vi "PH_Beckhoff_Application.declare digital PILS external OutputTags.vi"() -> (0 "Digital Outputs":T2, 1 "Description":string)   [LabVIEW 2014, in "PH_Beckhoff_Application.lvlib"]
uses:
  PH_Beckhoff_Application.lvlib
  PH_Beckhoff/PH_Beckhoff.Digital Outputs.ctl
  PH_Beckhoff/PH_Beckhoff.lvlib
panel:
  in  "Digital Output Value":T1
  out "Right Size?":bool
  # "Let this VI run to check the size!"
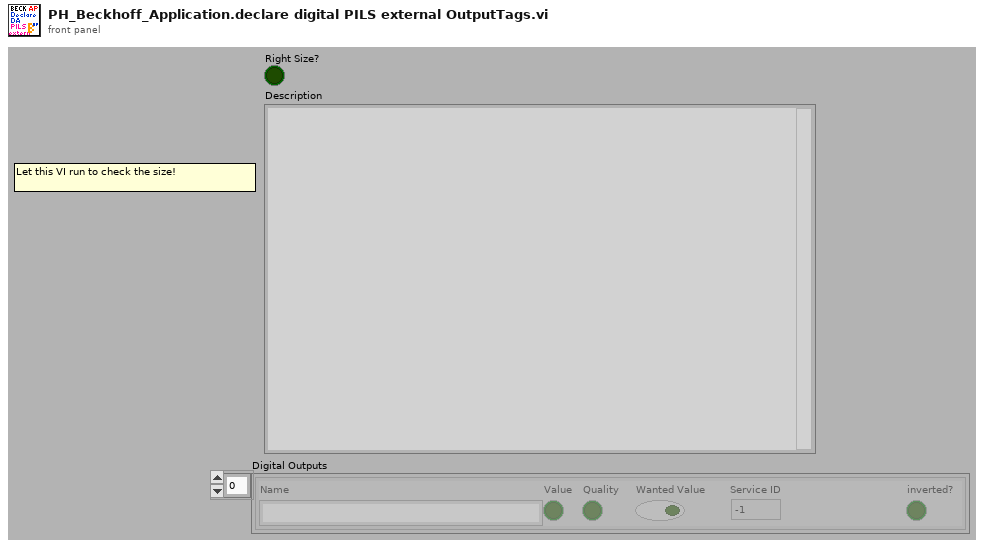
[diagram p1: front panel]
types:
  T1 = cluster{"Name":string, "Value":bool, "Quality":bool, "Wanted Value":bool, "Service ID":i32, "inverted?":bool}
  T2 = typedef "PH_Beckhoff.lvlib/PH_Beckhoff.Digital Outputs.ctl" = cluster{"Name":string, "Value":bool, "Quality":bool, "Wanted Value":bool, "Service ID":i32, "inverted?":bool}[]
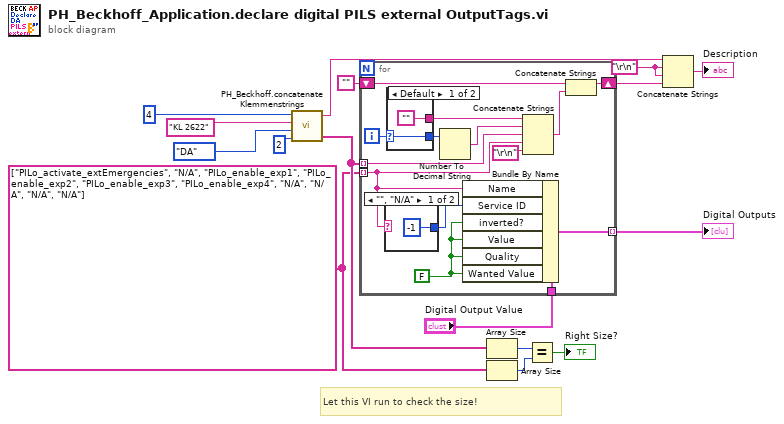
[diagram p0: block diagram]
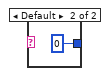
[diagram p2: hidden frame]
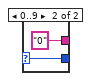
[diagram p3: hidden frame]
diagram:
  w1 = string[] ["PILo_activate_extEmergencies", "N/A", "PILo_enable_exp1", "PILo_enable_exp2", "PILo_enable_exp3", "PILo_enable_exp4", "N/A", "N/A", "N/A", "N/A"] ("Array")
  w15 = "\r\n"
  # "Let this VI run to check the size!"
  n1 = call "PH_Beckhoff.concatenate Klemmenstrings.vi"("# of In- or Outputs"=2, "Type"=enum16{"AE", "AA", "DE", "DA"}."DA", "Klemmenname"="KL 2622", "Quantity"=4 ("size(s)")) -> ("concatenated string array"=w2:string[], "\"<Type>: <Quantity> x <Klemmenname>\""=w3:string)  [unwired: 1 out]
  n2 = for {
    tunnel: w1 -> [w21] mode=indexing
    tunnel: w2 -> [w26] mode=indexing
    shift-right: [w24] -> w8
    shift-left: "" -> [w23]
    tunnel: "Digital Output Value" -> [w22]
    tunnel: [w19] -> w4 mode=indexing
    i -> [w30]
    w18 = FALSE ("Quality")
    n3 = case shown="\"\", \"N/A\"" w21 {
      tunnel: [-1 0] -> w20
      frame "", "N/A" {
      }
      frame Default {
      }
    }
    n4 = case shown="Default" w30 {
      selector: w30 -> [w33 w36]
      tunnel: [w33 w36] -> w29
      tunnel: ["" "0"] -> w28
      frame Default {
      }
      frame 0..9 {
      }
    }
    n5 = Number To Decimal String(number=w29) -> (decimal integer string=w27:string)  [unwired: 1 in]
    n6 = Bundle By Name(cluster=w22, "Name"=w21, "Service ID"=w20, "inverted?"=w18, "Value"=w18, "Quality"=w18, "Wanted Value"=w18) -> (w19:T1)
    n7 = Concatenate Strings(w28, w27, w26, w21, "\r\n") -> (w25:string)
    n8 = Concatenate Strings(w23, w25) -> (w24:string)
  }
  "Digital Outputs" <- w4
  n9 = Array Size(array=w2) -> (size(s)=w11:i32)
  n10 = Array Size(array=w1) -> (size(s)=w7:i32)
  n11 = Equal?(x=w11, y=w7) -> (x = y?=→"Right Size?":bool)
  n12 = Concatenate Strings(w3, w15, w15, w8) -> (→"Description":string)
